vi "startUp.vi"(8 "error in (no error)":errorcluster, 10 "ScriptEvent":refnum<class "ScriptEvent.lvclass">, 11 "Rf_Ramp_Action in":refnum<class "Rf_Ramp_Action.lvclass">) -> (0 "error out":errorcluster, 3 "Rf_Ramp_Action out":refnum<class "Rf_Ramp_Action.lvclass">)   [LabVIEW 2011, in "Views.lvlib" / "ScriptEditor.lvlib" / "Rf_Ramp_Action.lvclass"]
uses:
  Rf_Ramp_Action.lvclass
  Tools/Scripting/ScriptingEvent/ScriptEvent.lvclass
  Tools/Scripting/ScriptingEvent/ScriptEvents/RfRamp/RfRamp.lvclass
  Rf_Ramp_Action.lvclass/Rf_Ramp_Action.ctl
  ActionPanel.lvclass
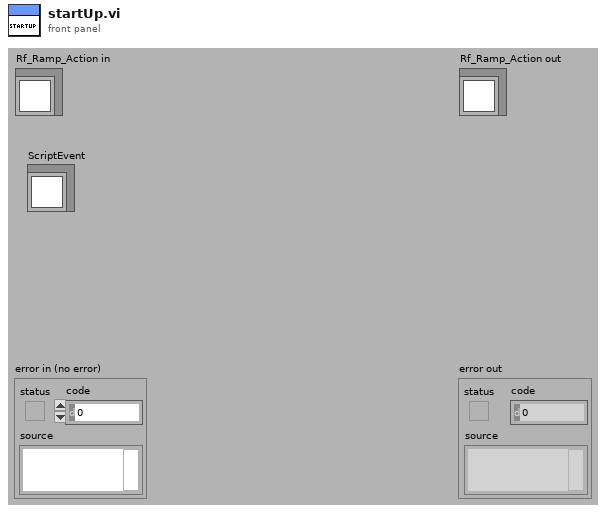
[diagram p1: front panel]
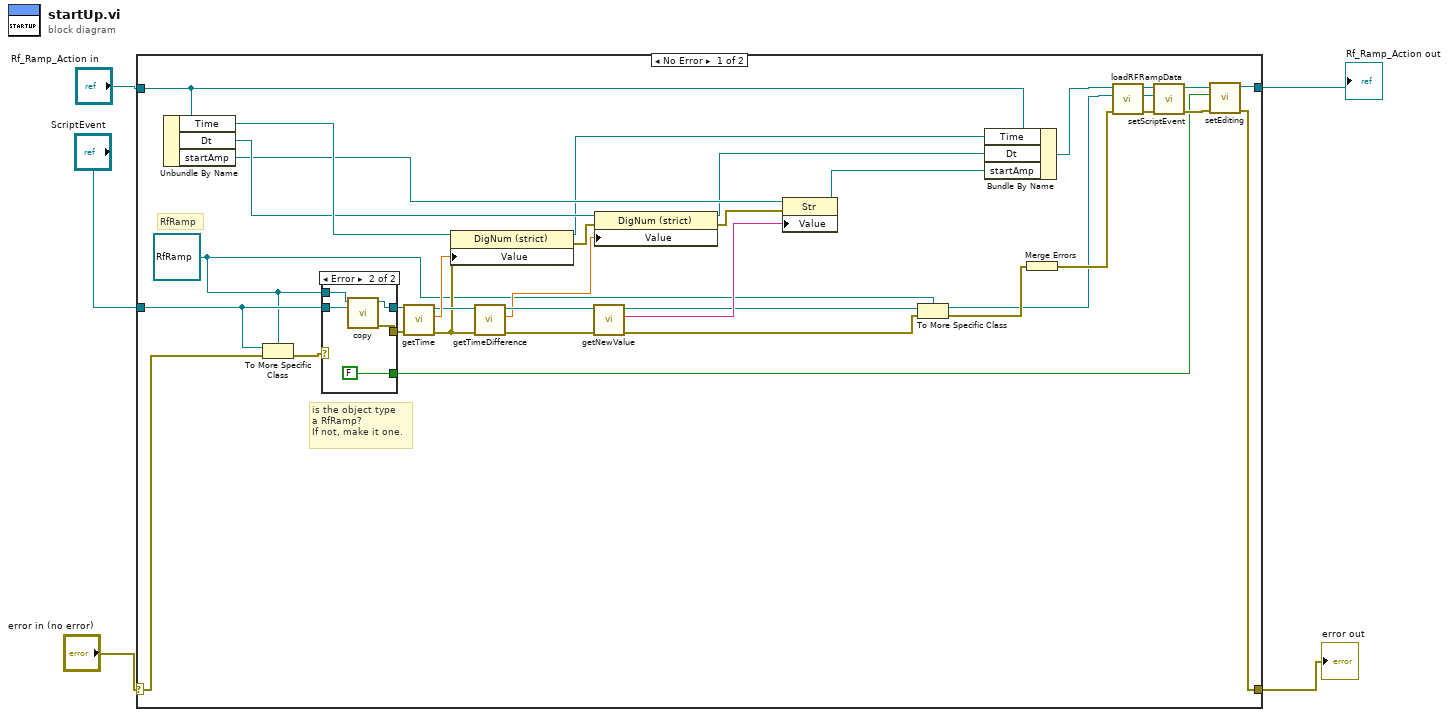
[diagram p0: block diagram]
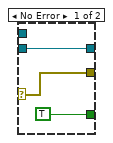
[diagram p2: hidden frame]
diagram:
  n1 = case shown="No Error" "error in (no error)" {
    selector: "error in (no error)" -> [w22 w51]
    tunnel: [w18 w51] -> w2
    tunnel: [w20 w50] -> w3
    tunnel: "Rf_Ramp_Action in" -> [w16 w50]
    tunnel: "ScriptEvent" -> [w38 _]
    frame No Error {
      w12 = refnum<class "RfRamp.lvclass"> refnum ("Tools.lvlib:Scripting.lvlib:RfRamp.lvclass")
      # "RfRamp"
      # "is the object type\na RfRamp?\nIf not, make it one."
      n2 = Unbundle By Name(w16) -> ("Time"=w37:refnum<vi>, "Dt"=w36:refnum<vi>, "startAmp"=w35:refnum<vi>)
      n3 = To More Specific Class(target class=w12, reference=w38, error in=w22) -> (error out=w41:errorcluster)  [unwired: 1 out]
      n4 = case shown="Error" w41 {
        selector: w41 -> [w43 _]
        tunnel: w38 -> [w44 w48]
        tunnel: w12 -> [_ w49]
        tunnel: [w43 w47] -> w40
        tunnel: [w44 w46] -> w39
        tunnel: [TRUE FALSE] -> w17
        frame No Error {
        }
        frame Error {
          n5 = call-dynamic "copy.vi"("ScriptEventForCopy"=w48, "RfRamp in"=w49) -> ("error out"=w47:errorcluster, "RfRamp out"=w46:refnum<class "RfRamp.lvclass">)  [unwired: 8 in]
        }
      }
      n6 = call "getTime.vi"("error in (no error)"=w40, "ScriptEvent.lvclass in"=w39) -> ("error out"=w28:errorcluster, "time"=w34:dbl, "ScriptEvent.lvclass out"=w33:refnum<class "ScriptEvent.lvclass">)  [unwired: 7 in]
      n7 = property class="DigNum (strict)"(reference=w37, error in=w28, "Value"=w34) -> (reference out=w25:refnum<vi>, error out=w27:errorcluster)
      n8 = call "getTimeDifference.vi"("error in (no error)"=w28, "ScriptEvent.lvclass in"=w33) -> ("error out"=w29:errorcluster, "time difference"=w31:dbl, "ScriptEvent.lvclass out"=w32:refnum<class "ScriptEvent.lvclass">)  [unwired: 7 in]
      n9 = call "getNewValue.vi"("error in (no error)"=w29, "ScriptEvent.lvclass in"=w32) -> ("error out"=w14:errorcluster, "newValue"=w30:string, "ScriptEvent.lvclass out"=w15:refnum<class "ScriptEvent.lvclass">)  [unwired: 7 in]
      n10 = property class="DigNum (strict)"(reference=w36, error in=w27, "Value"=w31) -> (reference out=w24:refnum<vi>, error out=w26:errorcluster)
      n11 = property class="Str"(reference=w35, error in=w26, "Value"=w30) -> (reference out=w13:refnum<vi>)  [unwired: 1 out]
      n12 = To More Specific Class(target class=w12, reference=w15, error in=w14) -> (specific class reference=w6:refnum<class "RfRamp.lvclass">, error out=w23:errorcluster)
      n13 = Bundle By Name(cluster=w16, "Time"=w25, "Dt"=w24, "startAmp"=w13) -> (w11:refnum<class "Rf_Ramp_Action.lvclass">)
      n14 = Merge Errors(w23) -> (w7:errorcluster)
      n15 = call "loadRFRampData.vi"("error in (no error)"=w7, "RfRamp"=w6, "Rf_Ramp_Action in"=w11) -> ("error out"=w8:errorcluster, "RfRamp out"=w9:refnum<class "RfRamp.lvclass">, "Rf_Ramp_Action out"=w10:refnum<class "Rf_Ramp_Action.lvclass">)  [unwired: 6 in]
      n16 = call "setScriptEvent.vi"("error in (no error)"=w8, "ScriptEvent.lvclass"=w9, "ActionPanel.lvclass in"=w10) -> ("error out"=w19:errorcluster, "ActionPanel.lvclass out"=w21:refnum<class "Rf_Ramp_Action.lvclass">)  [unwired: 7 in]
      n17 = call "setEditing.vi"("error in (no error)"=w19, "editing?"=w17, "ActionPanel.lvclass in"=w21) -> ("error out"=w18:errorcluster, "ActionPanel.lvclass out"=w20:refnum<class "Rf_Ramp_Action.lvclass">)  [unwired: 7 in]
    }
    frame Error {
    }
  }
  "error out" <- w2
  "Rf_Ramp_Action out" <- w3
